vi "ASI_stage_main.vi"   [LabVIEW 2015]
uses:
  CONTROLS/Q_main_element.ctl
  CONTROLS/Q_ASI_stage_element.ctl
  GLOBAL/Global_ASI_stage.vi
  GLOBAL/Global_ABORT.vi
  GLOBAL/Global_MAIN.vi
types:
  T1 = typedef "Q_ASI_stage_element.ctl" = cluster{"variant":variant, "Instruction":enum16{"ASI_idle", "ASI_initialize", "ASI_error", "ASI_security_stop", "ASI_read_XYZ", "ASI_up", "ASI_down", "ASI_left", "ASI_right", "ASI_save_XY", "ASI_move_to_XY", "ASI_brightfield", "ASI_init_scan", "ASI_init_merFISH", "ASI_move_to_XY_merFISH", "ASI_move_to_Z_merFISH", "ASI_init_autofocus_search_merFISH", "ASI_close_autofocus_search_merFISH", "ASI_adjust_piezo_autofocus_merFISH", "ASI_set_piezo_autofocus_to_reference_position_merFISH_TL", "ASI_close_merFISH", "ASI_stop"}}
  T2 = typedef "Q_main_element.ctl" = cluster{"variant":variant, "Instruction":enum16{"Main_idle", "Main_initialize", "Main_initialize_TDMS", "Main_initialize_Queue", "Main_error", "Main_DAQ_initialization_results", "Main_ASI_initialization_results", "Main_Piezo_initialization_results", "Main_Valve_initialization_results", "Main_Pump_initialization_results", "Main_CAMERA_initialization_results", "Main_FPGA_initialization_results", "Main_DAQ_error", "Main_ASI_error", "Main_Piezo_error", "Main_CAMERA_error", "Main_Valve_error", "Main_Pump_error", "Main_FPGA_error", "Main_start_acquiring", "Main_not_acquiring", "Main_acquiring", "Main_stop_acquiring", "Main_change_exposure", "Main_change_z_scan_parameters", "Main_define_ROI", "Main_define_mosaic", "Main_read_kinetic_time", "Main_cooler", "Main_read_temperature", "Main_save_XY", "Main_load_XY", "Main_discard_XY", "Main_move_to_XY", "Main_measure_QPD", "Main_autofocus_calibration", "Main_autofocus_initialization", "Main_autofocus_stop", "Main_save_PID", "Main_change_H_valve_position", "Main_two_way_valve", "Main_save_movie", "Main_init_single_scan", "Main_single_scan", "Main_stop_single_scan", "Main_merFISH_illumination_parameters", "Main_merFISH_buffer_probe_list", "Main_merFISH_injections_procedure", "Main_merFISH_save_setpoint", "Main_merFISH_DAPI_parameters", "Main_merFISH_Brightfield_parameters", "Main_merFISH_save_embryo_ROI", "Main_merFISH_init", "Main_merFISH_resume", "Main_merFISH_start_autofocus", "Main_merFISH_open_close_valve_merFISH", "Main_merFISH_open_close_valve_photobleaching", "Main_merFISH_hybridization", "Main_merFISH_move_to_ROI", "Main_merFISH_wait_stabilization", "Main_merFISH_move_to_REF", "Main_merFISH_scan", "Main_merFISH_photobleaching_injection", "Main_merFISH_photobleaching", "Main_merFISH_send_email", "Main_merFISH_close", "Main_STOP"}}
  T3 = cluster{"XY ROI0":dbl[], "Brightfield intensity":dbl, "Illumination source":bool}
  T4 = enum16{"ASI_idle", "ASI_initialize", "ASI_error", "ASI_security_stop", "ASI_read_XYZ", "ASI_up", "ASI_down", "ASI_left", "ASI_right", "ASI_save_XY", "ASI_move_to_XY", "ASI_brightfield", "ASI_init_scan", "ASI_init_merFISH", "ASI_move_to_XY_merFISH", "ASI_move_to_Z_merFISH", "ASI_init_autofocus_search_merFISH", "ASI_close_autofocus_search_merFISH", "ASI_adjust_piezo_autofocus_merFISH", "ASI_set_piezo_autofocus_to_reference_position_merFISH_TL", "ASI_close_merFISH", "ASI_stop"}
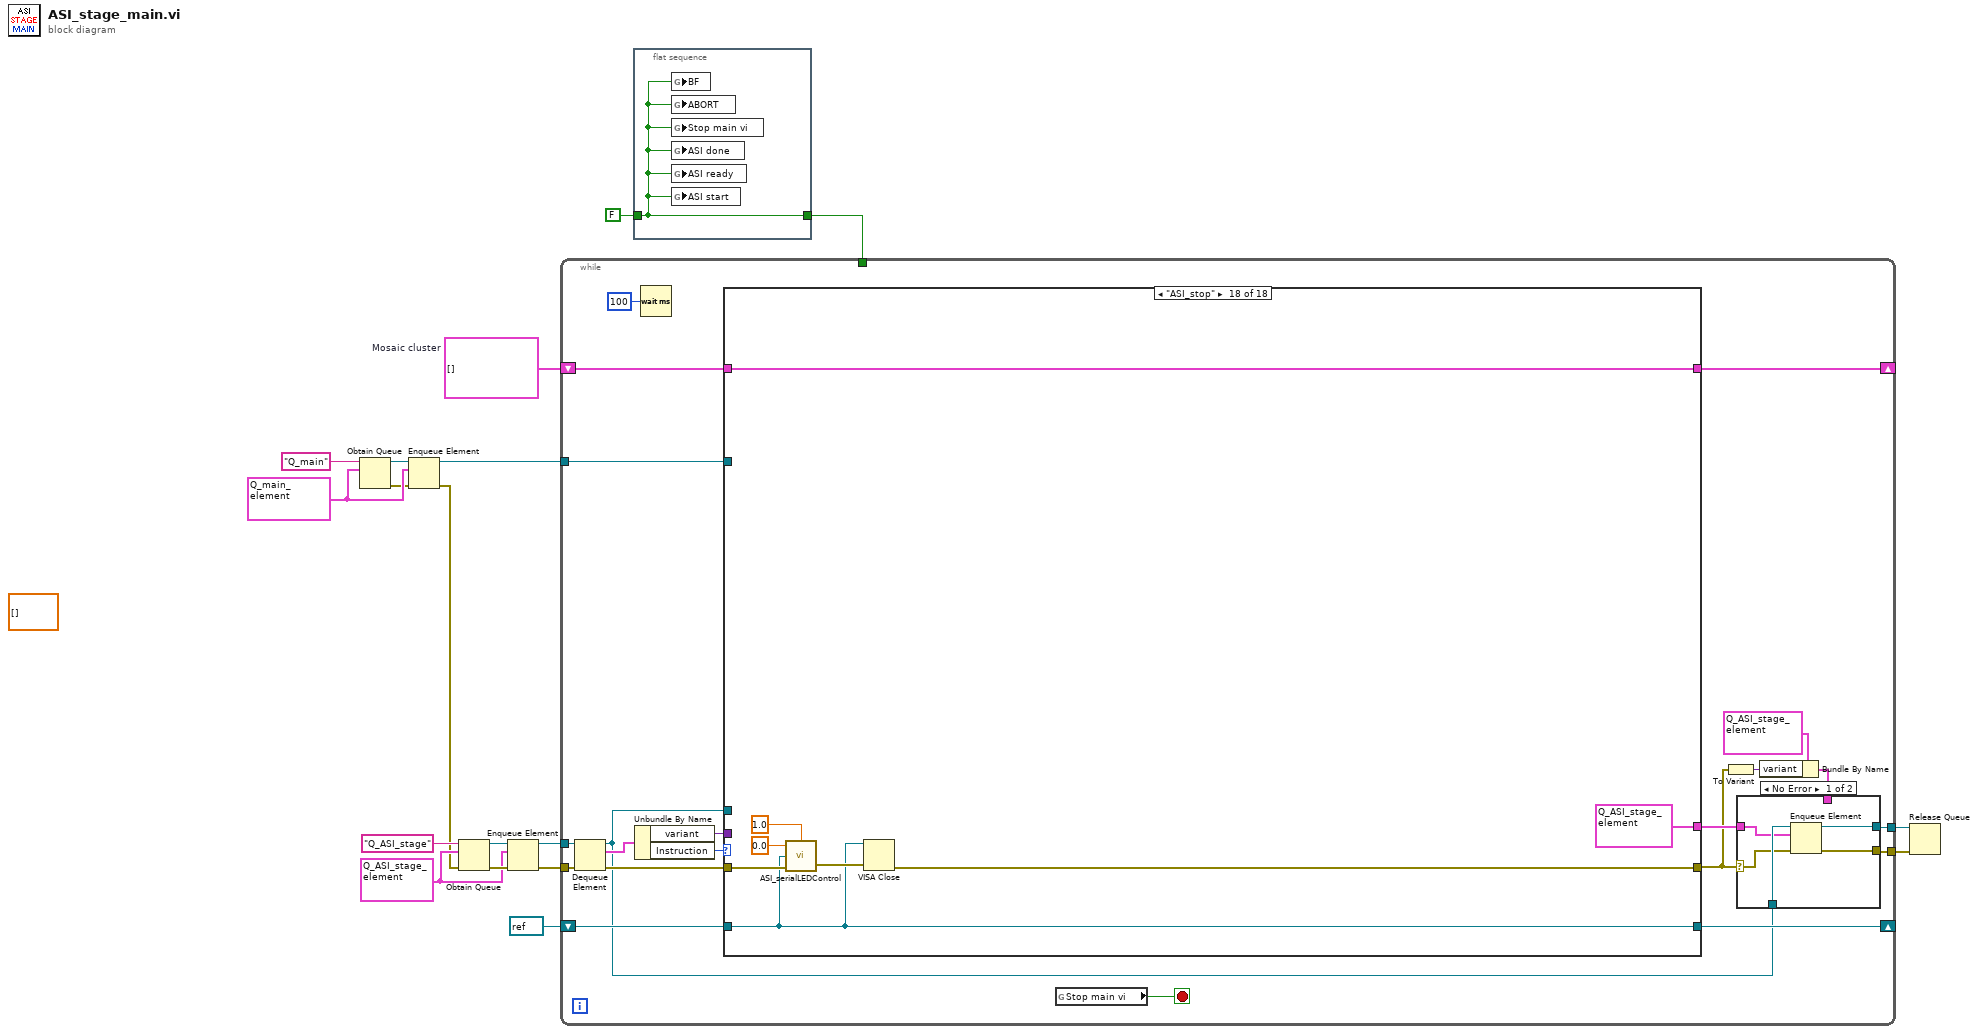
[diagram p0: block diagram]
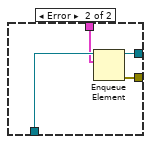
[diagram p2: hidden frame]
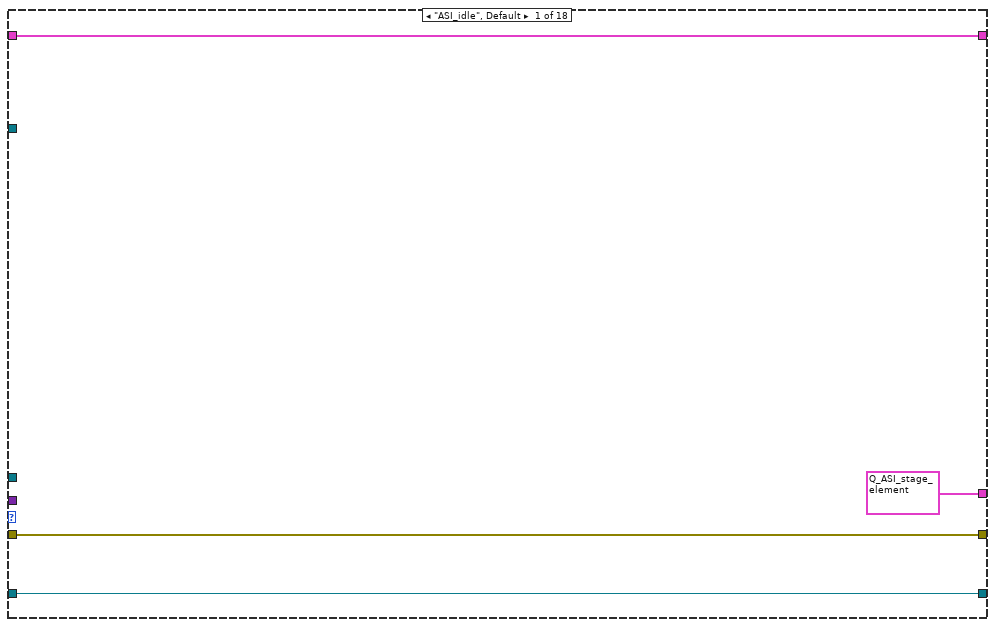
[diagram p3: hidden frame]
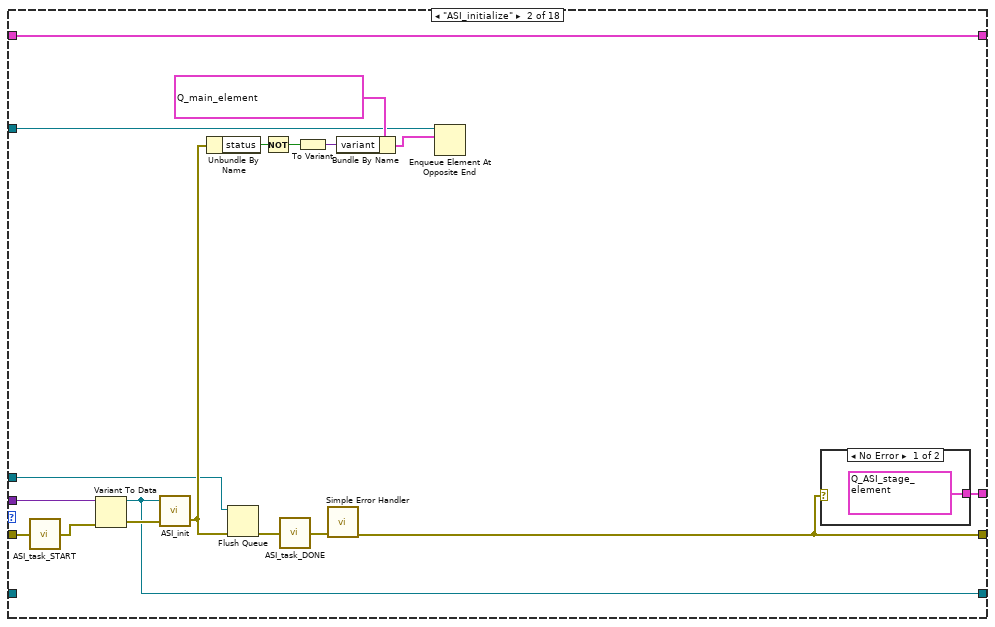
[diagram p4: hidden frame]
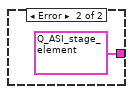
[diagram p5: hidden frame]
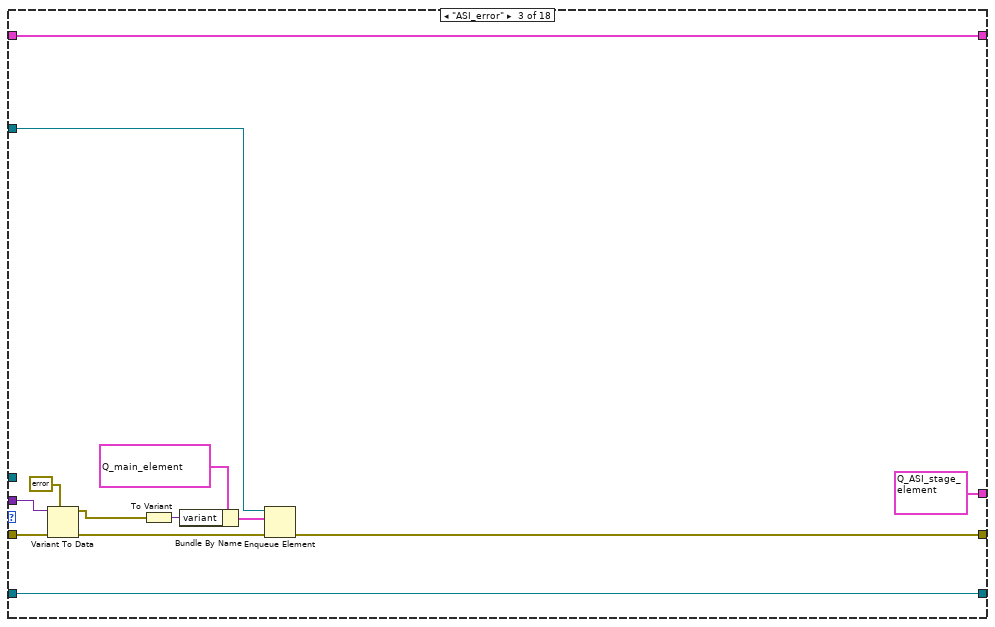
[diagram p6: hidden frame]
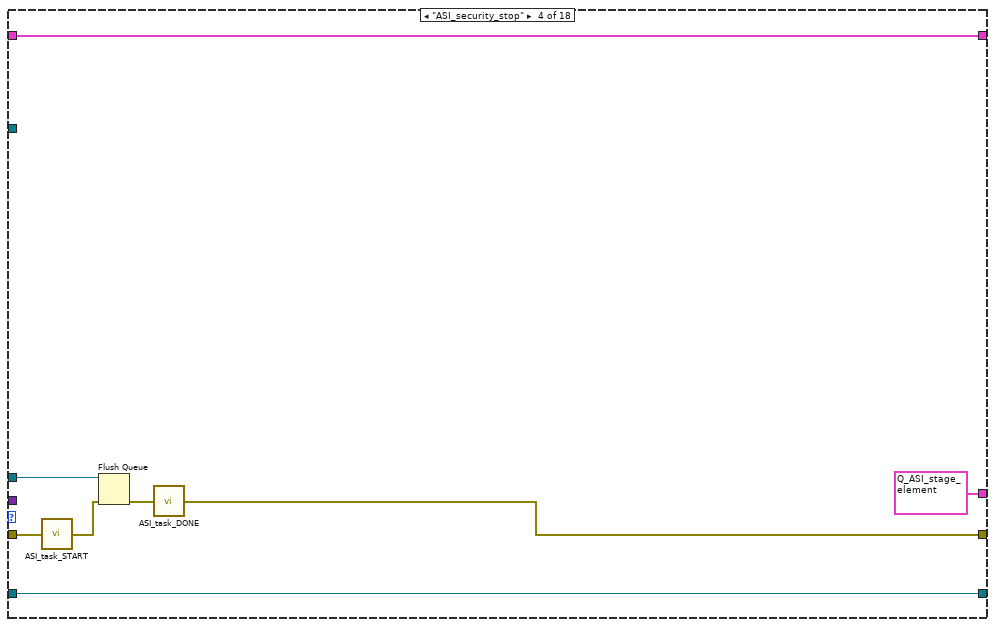
[diagram p7: hidden frame]
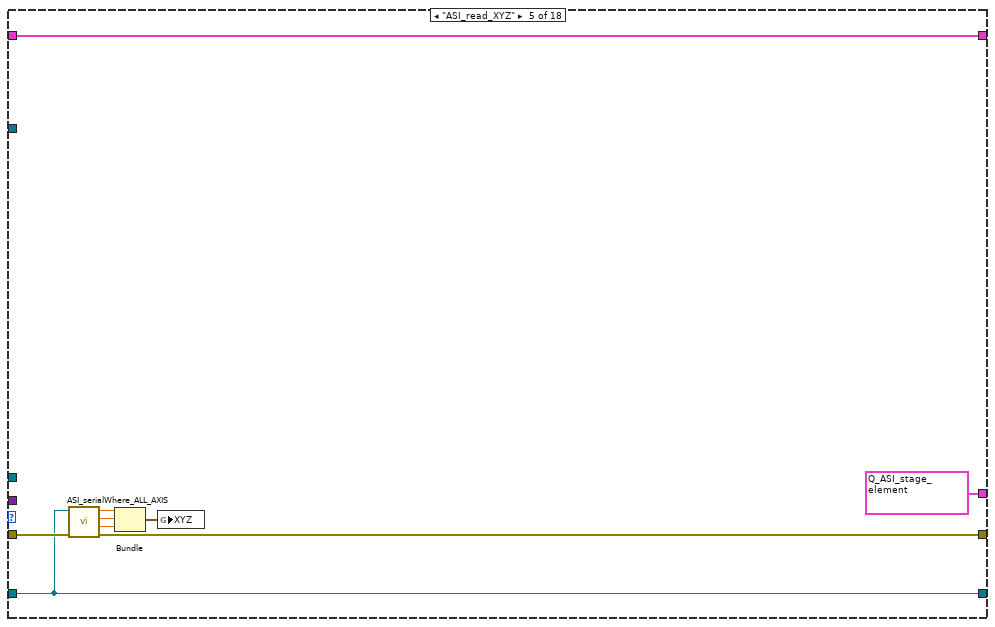
[diagram p8: hidden frame]
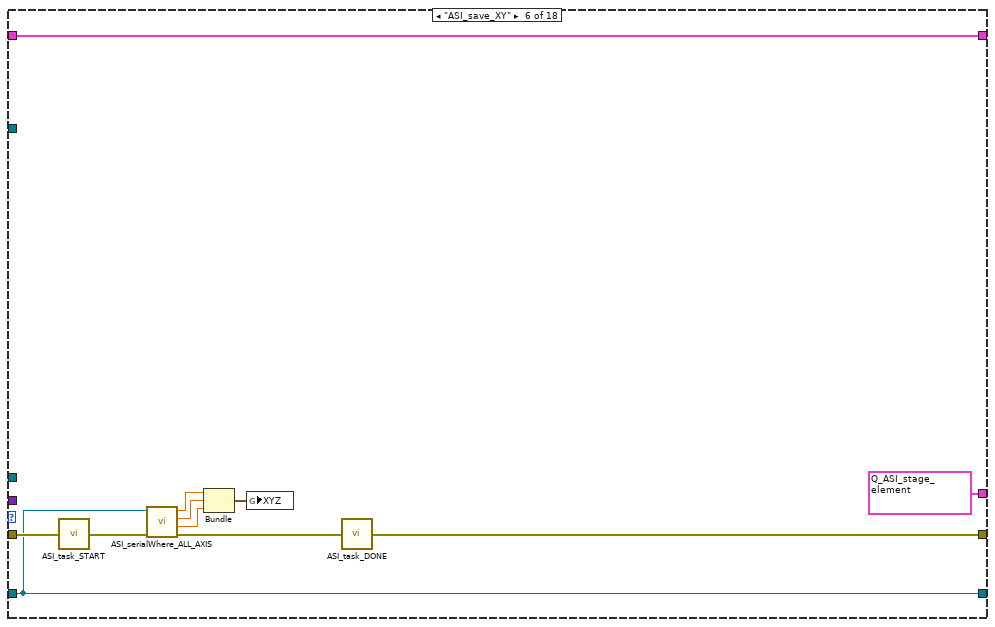
[diagram p9: hidden frame]
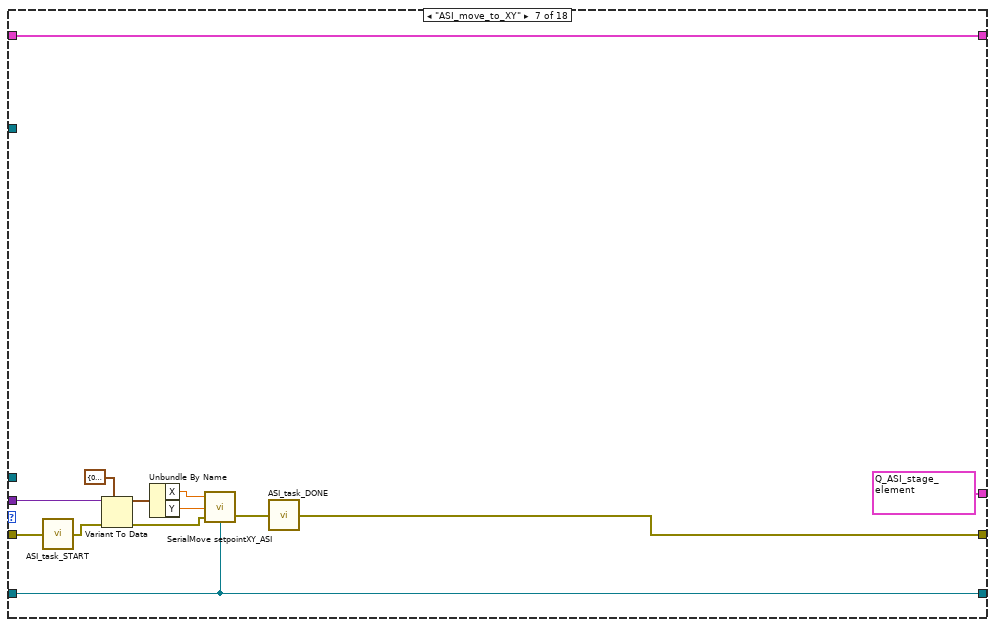
[diagram p10: hidden frame]
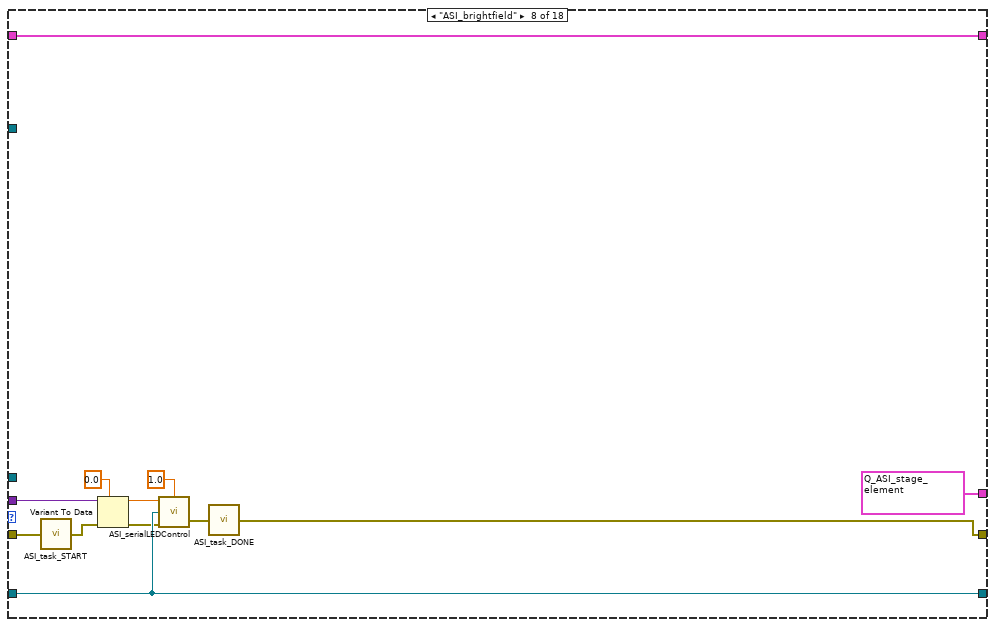
[diagram p11: hidden frame]
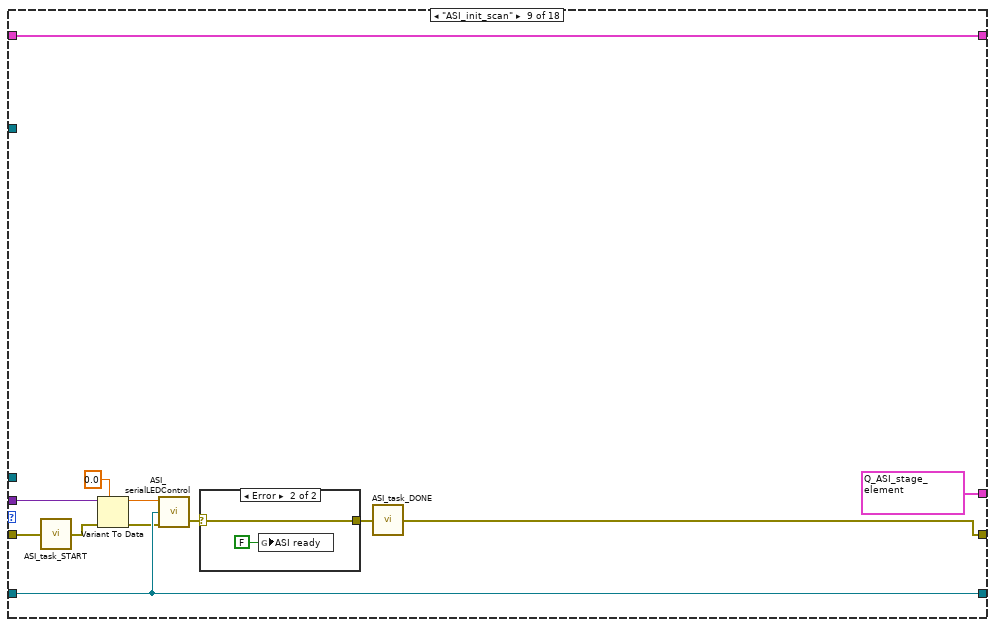
[diagram p12: hidden frame]
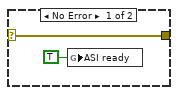
[diagram p13: hidden frame]
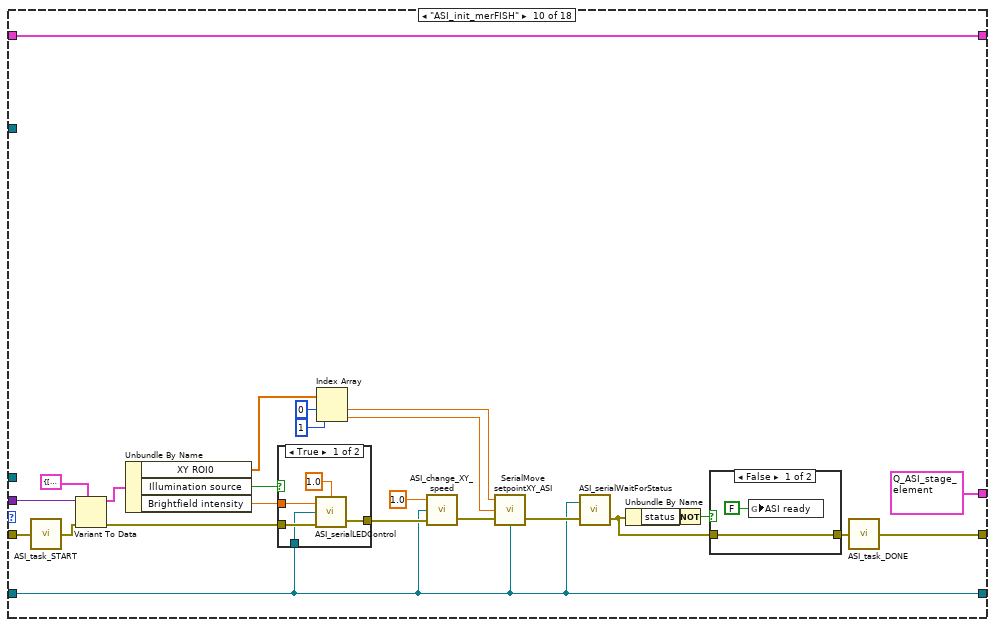
[diagram p14: hidden frame]
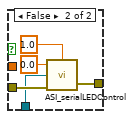
[diagram p15: hidden frame]
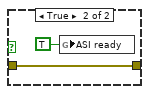
[diagram p16: hidden frame]
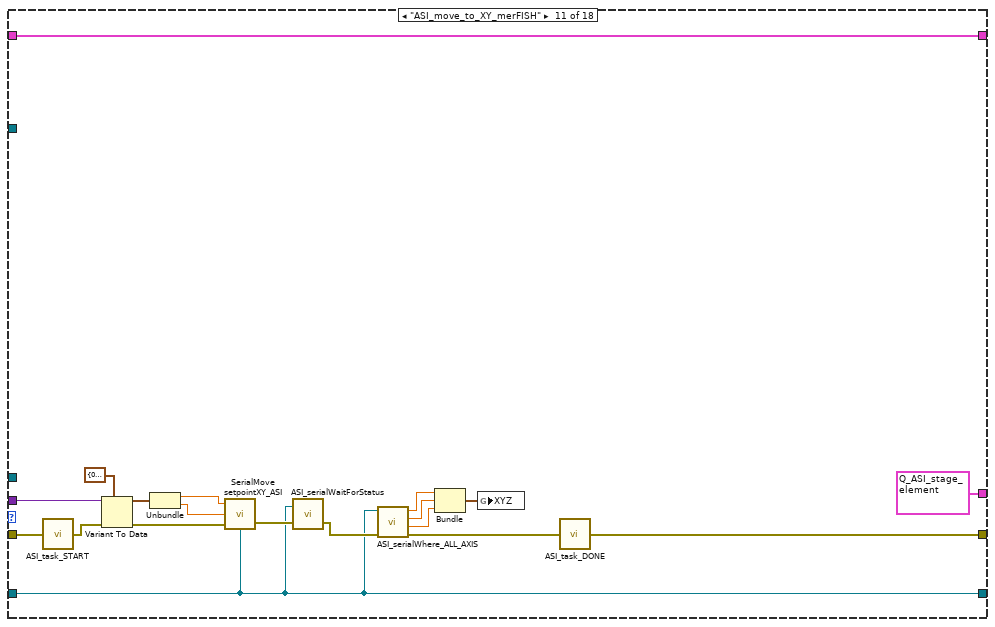
[diagram p17: hidden frame]
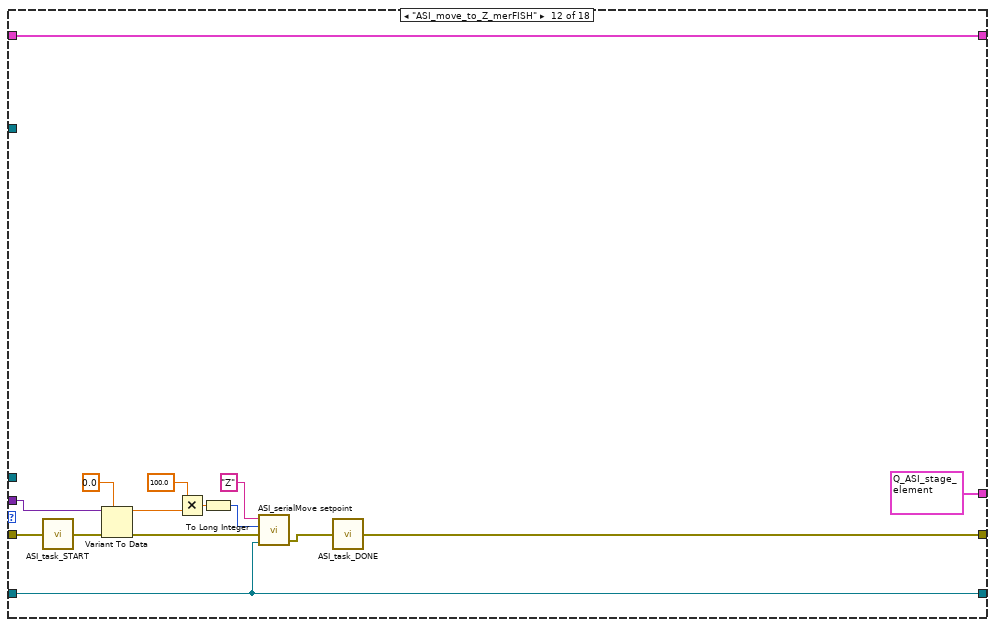
[diagram p18: hidden frame]
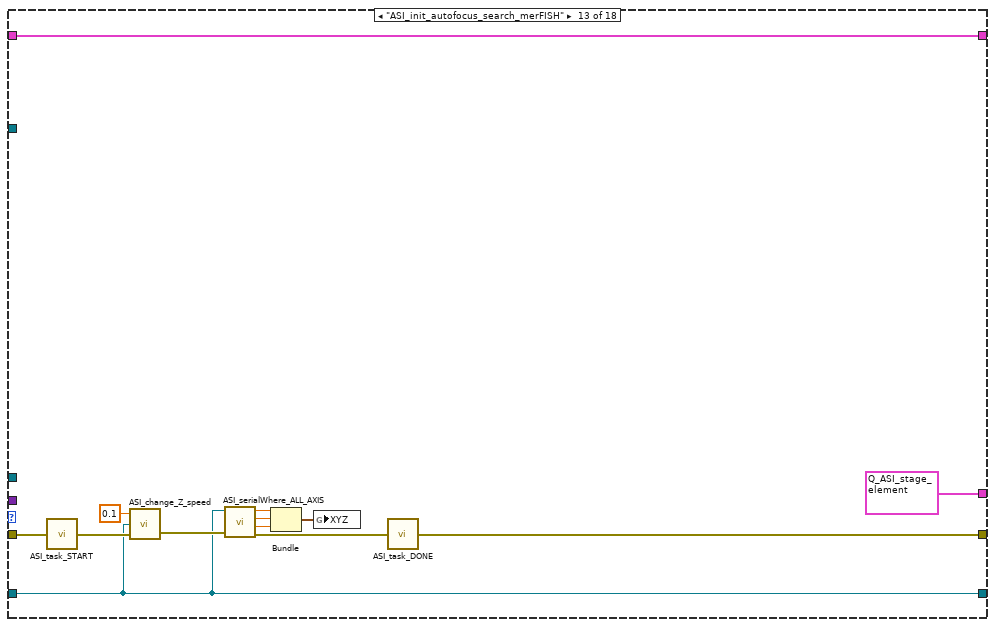
[diagram p19: hidden frame]
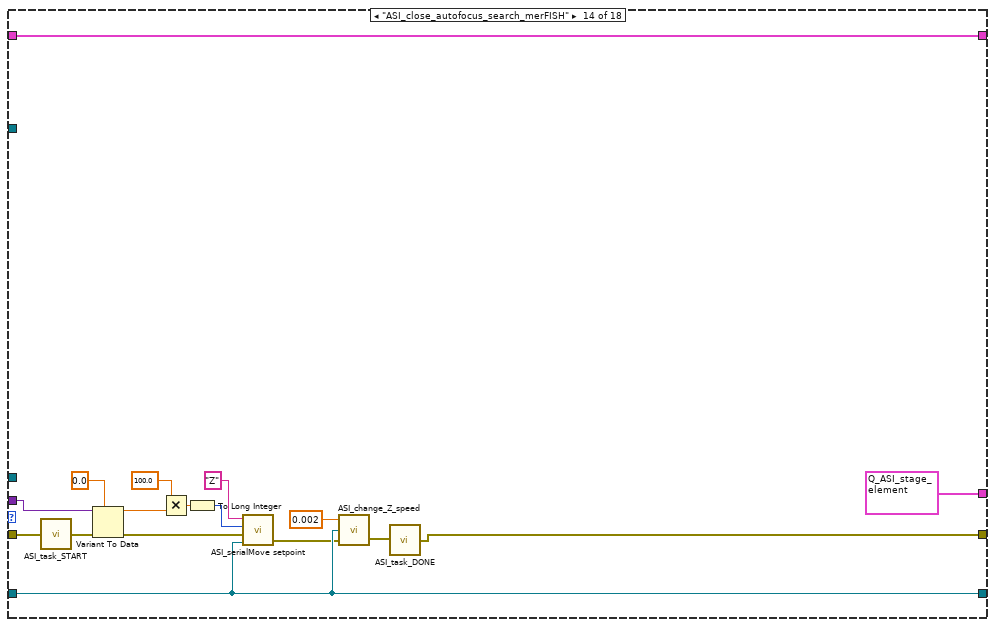
[diagram p20: hidden frame]
diagram:
  w1 = cluster{dbl[], dbl[]}[] []  # Mosaic cluster
  (unwired) dbl[][] [] ("XY positions 2")
  w4 = T1 {"variant"=variant, "Instruction"=enum."ASI_idle"} ("Q_ASI_stage")
  w11 = T2 {"variant"=variant, "Instruction"=enum."Main_idle"} ("Q_main_element")
  n1 = Obtain Queue(name (unnamed)="Q_main", element data type=w11) -> (queue out=w9:refnum<queue>, error out=w10:errorcluster)  [unwired: 3 in, 1 out]
  n2 = Enqueue Element(queue=w9, element=w11, error in (no error)=w10) -> (queue out=w7:refnum<queue>, error out=w2:errorcluster)  [unwired: 1 in, 1 out]
  n3 = Obtain Queue(name (unnamed)="Q_ASI_stage", element data type=w4, error in (no error)=w2) -> (queue out=w17:refnum<queue>, error out=w16:errorcluster)  [unwired: 2 in, 1 out]
  n4 = Enqueue Element(queue=w17, element=w4, error in (no error)=w16) -> (queue out=w15:refnum<queue>, error out=w14:errorcluster)  [unwired: 1 in, 1 out]
  n5 = while {
    tunnel: w15 -> [w38]
    tunnel: w14 -> [w37]
    tunnel: [w32] -> w13
    tunnel: [w31] -> w12
    tunnel: w7 -> [w30]
    tunnel: w5 -> [_]
    shift-right: [w26] -> _
    shift-left: refnum<visa-resource-name> refnum ("VISA resource name") -> [w27]
    shift-right: [w21] -> _
    shift-left: w1 -> [w20]
    stop <- w39 stop-if-true
    n6 = Dequeue Element(queue=w38, error in (no error)=w37) -> (queue out=w19:refnum<queue>, element=w36:T1, error out=w34:errorcluster)  [unwired: 1 in, 1 out]
    n7 = Unbundle By Name(w36) -> ("variant"=w29:variant, "Instruction"=w35:T4)
    n8 = Wait (ms)(milliseconds to wait=u32 100) -> ()  [unwired: 1 out]
    n9 = case shown="\"ASI_stop\"" w35 {
      tunnel: w34 -> [w52 w68 w80 w91 w102 w113 w126 w137 w149 w178 w212 w215 w240 w247 w262 w303 w331 w339]
      tunnel: [w52 w54 w74 w88 w101 w108 w121 w130 w142 w174 w207 w214 w234 w256 w259 w300 w330 w340] -> w22
      tunnel: [T1 {"variant"=variant, "Instruction"=enum."ASI_idle"} ("Q_ASI_stage") w70 T1 {"variant"=variant, "Instruction"=enum."ASI_idle"} ("Q_ASI_stage") T1 {"variant"=variant, "Instruction"=enum."ASI_idle"} ("Q_ASI_stage") T1 {"variant"=variant, "Instruction"=enum."ASI_read_XYZ"} ("Q_ASI_stage") T1 {"variant"=variant, "Instruction"=enum."ASI_read_XYZ"} ("Q_ASI_stage") T1 {"variant"=variant, "Instruction"=enum."ASI_read_XYZ"} ("Q_ASI_stage") T1 {"variant"=variant, "Instruction"=enum."ASI_read_XYZ"} ("Q_ASI_stage") T1 {"variant"=variant, "Instruction"=enum."ASI_read_XYZ"} ("Q_ASI_stage") T1 {"variant"=variant, "Instruction"=enum."ASI_idle"} ("Q_ASI_stage") T1 {"variant"=variant, "Instruction"=enum."ASI_idle"} ("Q_ASI_stage") T1 {"variant"=variant, "Instruction"=enum."ASI_idle"} ("Q_ASI_stage") T1 {"variant"=variant, "Instruction"=enum."ASI_idle"} ("Q_ASI_stage") T1 {"variant"=variant, "Instruction"=enum."ASI_idle"} ("Q_ASI_stage") T1 {"variant"=variant, "Instruction"=enum."ASI_idle"} ("Q_ASI_stage") T1 {"variant"=variant, "Instruction"=enum."ASI_idle"} ("Q_ASI_stage") T1 {"variant"=variant, "Instruction"=enum."ASI_read_XYZ"} ("Q_ASI_stage") T1 {"variant"=variant, "Instruction"=enum."ASI_stop"} ("Q_ASI_stage")] -> w33
      tunnel: w30 -> [_ w63 w77 _ _ _ _ _ _ _ _ _ _ _ _ _ _ _]
      tunnel: w29 -> [_ w69 w81 _ _ _ w125 w138 w150 w179 w211 w227 _ w246 w261 w304 _ _]
      tunnel: w19 -> [_ w57 _ w90 _ _ _ _ _ _ _ _ _ _ _ _ _ _]
      tunnel: w27 -> [w50 _ w84 w92 w99 w112 w116 w135 w147 w162 w195 w217 w230 w249 w260 w302 w326 w337]
      tunnel: [w50 w60 w84 w92 w99 w112 w116 w135 w147 w162 w195 w217 w230 w249 w260 w302 w326 w337] -> w26
      tunnel: [w49 w53 w73 w86 w94 w103 w114 w128 w139 w159 w194 w213 w228 w241 w258 w298 w321 w335] -> w21
      tunnel: w20 -> [w49 w53 w73 w86 w94 w103 w114 w128 w139 w159 w194 w213 w228 w241 w258 w298 w321 w335]
      frame "ASI_idle", Default {
      }
      frame "ASI_initialize" {
        n10 = call "ASI_task_START.vi"("error in"=w68) -> ("error out"=w56:errorcluster)
        n11 = Variant To Data(error in=w56, Variant=w69) -> (data=w60:refnum<visa-resource-name>, error out=w67:errorcluster)  [unwired: 1 in]
        n12 = call "ASI_init.vi"("error in (no error)"=w67, "VISA resource name"=w60) -> ("error out"=w59:errorcluster)  [unwired: 1 in, 1 out]
        n13 = Unbundle By Name(w59) -> ("status"=w62:bool)
        n14 = Flush Queue(queue=w57, error in (no error)=w59) -> (error out=w58:errorcluster)  [unwired: 2 out]
        n15 = Not(x=w62) -> (.not. x?=w61:bool)
        n16 = call "ASI_task_DONE.vi"("error in"=w58) -> ("error out"=w55:errorcluster)
        n17 = To Variant(anything=w61) -> (Variant=w65:variant)
        n18 = call <vilib>:"Simple Error Handler.vi"("error in (no error)"=w55) -> ("error out"=w54:errorcluster)  [unwired: 4 in, 4 out]
        n19 = Bundle By Name(cluster=T2 {"variant"=variant, "Instruction"=enum."Main_ASI_initialization_results"} ("element"), "variant"=w65) -> (w66:T2)
        n20 = Enqueue Element At Opposite End(queue=w63, element=w66) -> ()  [unwired: 2 in, 3 out]
        n21 = case shown="No Error" w54 {
          tunnel: [T1 {"variant"=variant, "Instruction"=enum."ASI_read_XYZ"} ("Q_ASI_stage") T1 {"variant"=variant, "Instruction"=enum."ASI_idle"} ("Q_ASI_stage")] -> w70
          frame No Error {
          }
          frame Error {
          }
        }
      }
      frame "ASI_error" {
        n22 = Variant To Data(error in=w80, type=errorcluster {"status"=FALSE, "code"=0, "source"=""} ("error out"), Variant=w81) -> (data=w75:errorcluster, error out=w76:errorcluster)
        n23 = To Variant(anything=w75) -> (Variant=w82:variant)
        n24 = Bundle By Name(cluster=T2 {"variant"=variant, "Instruction"=enum."Main_ASI_error"} ("Q_main_element"), "variant"=w82) -> (w78:T2)
        n25 = Enqueue Element(queue=w77, element=w78, error in (no error)=w76) -> (error out=w74:errorcluster)  [unwired: 1 in, 2 out]
      }
      frame "ASI_security_stop" {
        n26 = call "ASI_task_START.vi"("error in"=w91) -> ("error out"=w89:errorcluster)
        n27 = Flush Queue(queue=w90, error in (no error)=w89) -> (error out=w87:errorcluster)  [unwired: 2 out]
        n28 = call "ASI_task_DONE.vi"("error in"=w87) -> ("error out"=w88:errorcluster)
      }
      frame "ASI_read_XYZ" {
        n29 = call "ASI_serialWhere_ALL_AXIS.vi"("error in (no error)"=w102, "VISA resource name"=w99) -> ("error out"=w101:errorcluster, "Z"=w96:dbl, "Y"=w97:dbl, "X"=w98:dbl)  [unwired: 2 in]
        n30 = Bundle("X"=w98, "Y"=w97, "Z"=w96) -> (w95:cluster{"X":dbl, "Y":dbl, "Z":dbl})  [unwired: 1 in]
        n31 = global write "Global_ASI_stage.vi" "XYZ"(w95) -> ()
      }
      frame "ASI_save_XY" {
        n32 = call "ASI_task_START.vi"("error in"=w113) -> ("error out"=w110:errorcluster)
        n33 = call "ASI_serialWhere_ALL_AXIS.vi"("error in (no error)"=w110, "VISA resource name"=w112) -> ("error out"=w109:errorcluster, "Z"=w105:dbl, "Y"=w106:dbl, "X"=w107:dbl)  [unwired: 2 in]
        n34 = Bundle("X"=w107, "Y"=w106, "Z"=w105) -> (w104:cluster{"X":dbl, "Y":dbl, "Z":dbl})  [unwired: 1 in]
        n35 = global write "Global_ASI_stage.vi" "XYZ"(w104) -> ()
        n36 = call "ASI_task_DONE.vi"("error in"=w109) -> ("error out"=w108:errorcluster)
      }
      frame "ASI_move_to_XY" {
        n37 = call "ASI_task_START.vi"("error in"=w126) -> ("error out"=w124:errorcluster)
        n38 = Variant To Data(error in=w124, type=cluster{"X":dbl, "Y":dbl} {"X"=0.0, "Y"=0.0} ("output cluster"), Variant=w125) -> (data=w122:cluster{"X":dbl, "Y":dbl}, error out=w117:errorcluster)
        n39 = Unbundle By Name(w122) -> ("X"=w119:dbl, "Y"=w118:dbl)
        n40 = call "SerialMove setpointXY_ASI.vi"("VISA resource name"=w116, "error in"=w117, "Y"=w118, "X"=w119) -> ("error out"=w115:errorcluster)  [unwired: 1 in]
        n41 = call "ASI_task_DONE.vi"("error in"=w115) -> ("error out"=w121:errorcluster)
      }
      frame "ASI_brightfield" {
        n42 = call "ASI_task_START.vi"("error in"=w137) -> ("error out"=w131:errorcluster)
        n43 = Variant To Data(error in=w131, type=0.0 ("BF"), Variant=w138) -> (data=w132:dbl, error out=w133:errorcluster)
        n44 = call "ASI_serialLEDControl.vi"("Delay Time (s)"=1.0, "error in (no error)"=w133, "VISA resource name"=w135, "setpoint"=w132) -> ("error out"=w129:errorcluster)  [unwired: 1 out]
        n45 = call "ASI_task_DONE.vi"("error in"=w129) -> ("error out"=w130:errorcluster)
      }
      frame "ASI_init_scan" {
        n46 = call "ASI_task_START.vi"("error in"=w149) -> ("error out"=w143:errorcluster)
        n47 = Variant To Data(error in=w143, type=0.0 ("BF"), Variant=w150) -> (data=w144:dbl, error out=w145:errorcluster)
        n48 = call "ASI_serialLEDControl.vi"("error in (no error)"=w145, "VISA resource name"=w147, "setpoint"=w144) -> ("error out"=w141:errorcluster)  [unwired: 1 in, 1 out]
        n49 = case shown="Error" w141 {
          selector: w141 -> [w152 w154]
          tunnel: [w152 w154] -> w140
          frame No Error {
            n50 = global write "Global_ASI_stage.vi" "ASI ready"(TRUE ("ASI ready")) -> ()
          }
          frame Error {
            n51 = global write "Global_ASI_stage.vi" "ASI ready"(FALSE ("ASI ready")) -> ()
          }
        }
        n52 = call "ASI_task_DONE.vi"("error in"=w140) -> ("error out"=w142:errorcluster)
      }
      frame "ASI_init_merFISH" {
        n53 = call "ASI_task_START.vi"("error in"=w178) -> ("error out"=w175:errorcluster)
        n54 = Variant To Data(error in=w175, type=T3 {"XY ROI0"=[], "Brightfield intensity"=0.0, "Illumination source"=FALSE} ("output cluster"), Variant=w179) -> (data=w172:T3, error out=w176:errorcluster)
        n55 = Unbundle By Name(w172) -> ("XY ROI0"=w156:dbl[], "Illumination source"=w155:bool, "Brightfield intensity"=w171:dbl)
        n56 = case shown="True" w155 {
          tunnel: w176 -> [w184 w189]
          tunnel: w171 -> [w183 _]
          tunnel: [w182 w188] -> w166
          tunnel: w162 -> [w181 w187]
          frame True {
            n57 = call "ASI_serialLEDControl.vi"("Delay Time (s)"=1.0, "error in (no error)"=w184, "VISA resource name"=w181, "setpoint"=w183) -> ("error out"=w182:errorcluster)  [unwired: 1 out]
          }
          frame False {
            n58 = call "ASI_serialLEDControl.vi"("Delay Time (s)"=1.0, "error in (no error)"=w189, "VISA resource name"=w187, "setpoint"=0.0) -> ("error out"=w188:errorcluster)  [unwired: 1 out]
          }
        }
        n59 = Index Array(array=w156, index #1=0 ("index"), index #2=1 ("index")) -> (element #1=w168:dbl, element #2=w167:dbl)
        n60 = call "ASI_change_XY_speed.vi"("error in (no error)"=w166, "VISA resource name"=w162, "speed"=1.0) -> ("error out"=w164:errorcluster)  [unwired: 1 in]
        n61 = call "SerialMove setpointXY_ASI.vi"("VISA resource name"=w162, "error in"=w164, "Y"=w167, "X"=w168) -> ("error out"=w163:errorcluster)  [unwired: 1 in]
        n62 = call "ASI_serialWaitForStatus.vi"("error in"=w163, "VISA resource name"=w162) -> ("error out"=w160:errorcluster)  [unwired: 1 in]
        n63 = Unbundle By Name(w160) -> ("status"=w161:bool)
        n64 = Not(x=w161) -> (.not. x?=w158:bool)
        n65 = case shown="False" w158 {
          tunnel: [w190 w192] -> w173
          tunnel: w160 -> [w190 w192]
          frame False {
            n66 = global write "Global_ASI_stage.vi" "ASI ready"(FALSE ("ASI ready")) -> ()
          }
          frame True {
            n67 = global write "Global_ASI_stage.vi" "ASI ready"(TRUE ("ASI ready")) -> ()
          }
        }
        n68 = call "ASI_task_DONE.vi"("error in"=w173) -> ("error out"=w174:errorcluster)
      }
      frame "ASI_move_to_XY_merFISH" {
        n69 = call "ASI_task_START.vi"("error in"=w212) -> ("error out"=w210:errorcluster)
        n70 = Variant To Data(error in=w210, type=cluster{dbl, dbl} {0.0, 0.0} ("output cluster"), Variant=w211) -> (data=w208:cluster{dbl, dbl}, error out=w200:errorcluster)
        n71 = Unbundle(w208) -> (w198:dbl, w199:dbl)
        n72 = call "SerialMove setpointXY_ASI.vi"("VISA resource name"=w195, "error in"=w200, "Y"=w199, "X"=w198) -> ("error out"=w197:errorcluster)  [unwired: 1 in]
        n73 = call "ASI_serialWaitForStatus.vi"("error in"=w197, "VISA resource name"=w195) -> ("error out"=w196:errorcluster)  [unwired: 1 in]
        n74 = call "ASI_serialWhere_ALL_AXIS.vi"("error in (no error)"=w196, "VISA resource name"=w195) -> ("error out"=w205:errorcluster, "Z"=w202:dbl, "Y"=w203:dbl, "X"=w204:dbl)  [unwired: 2 in]
        n75 = Bundle("X"=w204, "Y"=w203, "Z"=w202) -> (w201:cluster{"X":dbl, "Y":dbl, "Z":dbl})  [unwired: 1 in]
        n76 = global write "Global_ASI_stage.vi" "XYZ"(w201) -> ()
        n77 = call "ASI_task_DONE.vi"("error in"=w205) -> ("error out"=w207:errorcluster)
      }
      frame "ASI_move_to_Z_merFISH" {
        n78 = call "ASI_task_START.vi"("error in"=w215) -> ("error out"=w226:errorcluster)
        n79 = Variant To Data(error in=w226, type=0.0, Variant=w227) -> (data=w218:dbl, error out=w219:errorcluster)
        n80 = Multiply(x=100.0, y=w218) -> (x*y=w221:dbl)
        n81 = To Long Integer(number=w221) -> (32bit integer=w220:i32)
        n82 = call "ASI_serialMove setpoint.vi"("Axis"="Z", "setpoint"=w220, "error in (no error)"=w219, "VISA resource name"=w217) -> ("error out"=w216:errorcluster)  [unwired: 3 in]
        n83 = call "ASI_task_DONE.vi"("error in"=w216) -> ("error out"=w214:errorcluster)
      }
      frame "ASI_init_autofocus_search_merFISH" {
        n84 = call "ASI_task_START.vi"("error in"=w240) -> ("error out"=w232:errorcluster)
        n85 = call "ASI_change_Z_speed.vi"("error in (no error)"=w232, "VISA resource name"=w230, "speed"=0.1) -> ("error out"=w231:errorcluster)  [unwired: 1 out]
        n86 = call "ASI_serialWhere_ALL_AXIS.vi"("error in (no error)"=w231, "VISA resource name"=w230) -> ("error out"=w233:errorcluster, "Z"=w236:dbl, "Y"=w237:dbl, "X"=w238:dbl)  [unwired: 2 in]
        n87 = Bundle("X"=w238, "Y"=w237, "Z"=w236) -> (w235:cluster{"X":dbl, "Y":dbl, "Z":dbl})  [unwired: 1 in]
        n88 = global write "Global_ASI_stage.vi" "XYZ"(w235) -> ()
        n89 = call "ASI_task_DONE.vi"("error in"=w233) -> ("error out"=w234:errorcluster)
      }
      frame "ASI_close_autofocus_search_merFISH" {
        n90 = call "ASI_task_START.vi"("error in"=w247) -> ("error out"=w242:errorcluster)
        n91 = Variant To Data(error in=w242, type=0.0 ("x"), Variant=w246) -> (data=w244:dbl, error out=w243:errorcluster)
        n92 = Multiply(x=100.0, y=w244) -> (x*y=w251:dbl)
        n93 = To Long Integer(number=w251) -> (32bit integer=w250:i32)
        n94 = call "ASI_serialMove setpoint.vi"("Axis"="Z", "setpoint"=w250, "error in (no error)"=w243, "VISA resource name"=w249) -> ("error out"=w248:errorcluster)  [unwired: 3 in]
        n95 = call "ASI_change_Z_speed.vi"("error in (no error)"=w248, "VISA resource name"=w249, "speed"=0.002) -> ("error out"=w254:errorcluster)  [unwired: 1 out]
        n96 = call "ASI_task_DONE.vi"("error in"=w254) -> ("error out"=w256:errorcluster)
      }
      frame "ASI_adjust_piezo_autofocus_merFISH" {
        # "In order to adjust the piezo position to 20um (when piezo position is below 10um)\nor 60um (when it is above 70um) without loosing the focus, \nthe ASI z position is changed here. Since the speed of the ASI stage movement\nis usually too fast, it is set to 2um/s and the backlash set to 1um."
        n97 = call "ASI_task_START.vi"("error in"=w262) -> ("error out"=w265:errorcluster)
        n98 = Variant To Data(error in=w265, type=cluster{"Min":dbl, "Max":dbl, "z":dbl} {"Min"=0.0, "Max"=0.0, "z"=0.0} ("Limits"), Variant=w261) -> (data=w269:cluster{"Min":dbl, "Max":dbl, "z":dbl}, error out=w263:errorcluster)
        n99 = Unbundle By Name(w269) -> ("Min"=w268:dbl, "z"=w267:dbl)
        n100 = Greater?(x=w268, y=w267) -> (0:w264:bool)
        n101 = case shown="True" w264 {
          tunnel: [w272 w285] -> w270
          tunnel: w260 -> [w281 w294]
          tunnel: w263 -> [w280 w293]
          tunnel: w267 -> [w277 w290]
          tunnel: w269 -> [w276 w287]
          frame True {
            n102 = Unbundle By Name(w276) -> ("Min"=w274:dbl)
            n103 = Add(x=w274, y=5.0) -> (x+y=w275:dbl)
            n104 = Subtract(x=w275, y=w277) -> (x-y=w284:dbl)
            n105 = Multiply(x=100.0, y=w284) -> (x*y=w279:dbl)
            n106 = To Long Integer(number=w279) -> (32bit integer=w278:i32)
            n107 = call "ASI_serialRelativeMove setpoint.vi"("VISA resource name"=w281, "error in (no error)"=w280, "setpoint"=w278, "Axis"="Z") -> ("error out"=w272:errorcluster)  [unwired: 1 in]
          }
          frame False {
            n108 = Unbundle By Name(w287) -> ("Max"=w289:dbl)
            n109 = Subtract(x=w289, y=5.0) -> (x-y=w286:dbl)
            n110 = Subtract(x=w286, y=w290) -> (x-y=w297:dbl)
            n111 = Multiply(x=100.0, y=w297) -> (x*y=w292:dbl)
            n112 = To Long Integer(number=w292) -> (32bit integer=w291:i32)
            n113 = call "ASI_serialRelativeMove setpoint.vi"("VISA resource name"=w294, "error in (no error)"=w293, "setpoint"=w291, "Axis"="Z") -> ("error out"=w285:errorcluster)  [unwired: 1 in]
          }
        }
        n114 = call "ASI_task_DONE.vi"("error in"=w270) -> ("error out"=w259:errorcluster)
      }
      frame "ASI_set_piezo_autofocus_to_reference_position_merFISH_TL" {
        # "In order to adjust the piezo position to 20um (when piezo position is below 10um)\nor 60um (when it is above 70um) without loosing the focus, \nthe ASI z position is changed here. Since the speed of the ASI stage movement\nis usually too fast, it is set to 2um/s and the backlash set to 1um."
        n115 = call "ASI_task_START.vi"("error in"=w303) -> ("error out"=w316:errorcluster)
        n116 = call "ASI_change_Z_speed.vi"("error in (no error)"=w316, "VISA resource name"=w302, "speed"=0.001) -> ("error out"=w299:errorcluster)  [unwired: 1 out]
        n117 = Variant To Data(error in=w299, type=cluster{"Ref":dbl, "z":dbl} {"Ref"=0.0, "z"=0.0} ("Limits"), Variant=w304) -> (data=w308:cluster{"Ref":dbl, "z":dbl}, error out=w305:errorcluster)
        n118 = Unbundle By Name(w308) -> ("Ref"=w314:dbl, "z"=w307:dbl)
        n119 = Subtract(x=w314, y=w307) -> (x-y=w309:dbl)
        n120 = Multiply(x=100.0, y=w309) -> (x*y=w312:dbl)
        n121 = To Long Integer(number=w312) -> (32bit integer=w313:i32)
        n122 = call "ASI_serialRelativeMove setpoint.vi"("VISA resource name"=w302, "error in (no error)"=w305, "setpoint"=w313, "Axis"="Z") -> ("error out"=w317:errorcluster)  [unwired: 1 in]
        n123 = call "ASI_change_Z_speed.vi"("error in (no error)"=w317, "VISA resource name"=w302, "speed"=0.5) -> ("error out"=w318:errorcluster)  [unwired: 1 out]
        n124 = call "ASI_task_DONE.vi"("error in"=w318) -> ("error out"=w300:errorcluster)
      }
      frame "ASI_close_merFISH" {
        n125 = call "ASI_task_START.vi"("error in"=w331) -> ("error out"=w329:errorcluster)
        n126 = call "ASI_serialLEDControl.vi"("Delay Time (s)"=1.0, "error in (no error)"=w329, "VISA resource name"=w326, "setpoint"=0.0) -> ("error out"=w327:errorcluster)  [unwired: 1 out]
        n127 = call "ASI_change_XY_speed.vi"("error in (no error)"=w327, "VISA resource name"=w326, "speed"=7.0) -> ("error out"=w324:errorcluster)  [unwired: 1 in]
        n128 = flat-sequence {
          tunnel: w324 -> [w333]
          tunnel: [w333] -> w323
          frame #0 {
            n129 = global write "Global_ASI_stage.vi" "ASI ready"(FALSE ("ASI ready")) -> ()
          }
        }
        n130 = call "ASI_task_DONE.vi"("error in"=w323) -> ("error out"=w330:errorcluster)
      }
      frame "ASI_stop" {
        n131 = call "ASI_serialLEDControl.vi"("Delay Time (s)"=1.0, "error in (no error)"=w339, "VISA resource name"=w337, "setpoint"=0.0) -> ("error out"=w338:errorcluster)  [unwired: 1 out]
        n132 = VISA Close(VISA resource name=w337, error in (no error)=w338) -> (error out=w340:errorcluster)
      }
    }
    n133 = global read "Global_MAIN.vi" "Stop main vi"() -> (w39:bool)
    n134 = To Variant(anything=w22) -> (Variant=w23:variant)
    n135 = Bundle By Name(cluster=T1 {"variant"=variant, "Instruction"=enum."ASI_error"} ("Q_ASI_stage"), "variant"=w23) -> (w24:T1)
    n136 = case shown="No Error" w22 {
      selector: w22 -> [w41 _]
      tunnel: w33 -> [w40 _]
      tunnel: [w44 w48] -> w32
      tunnel: [w43 w47] -> w31
      tunnel: w19 -> [w42 w46]
      tunnel: w24 -> [_ w45]
      frame No Error {
        n137 = Enqueue Element(queue=w42, element=w40, error in (no error)=w41) -> (queue out=w44:refnum<queue>, error out=w43:errorcluster)  [unwired: 1 in, 1 out]
      }
      frame Error {
        n138 = Enqueue Element(queue=w46, element=w45) -> (queue out=w48:refnum<queue>, error out=w47:errorcluster)  [unwired: 2 in, 1 out]
      }
    }
  }
  n139 = flat-sequence {
    tunnel: FALSE ("Stop main vi") -> [w342]
    tunnel: [w342] -> w5
    frame #0 {
      n140 = global write "Global_ASI_stage.vi" "BF"(w342) -> ()
      n141 = global write "Global_ABORT.vi" "ABORT"(w342) -> ()
      n142 = global write "Global_MAIN.vi" "Stop main vi"(w342) -> ()
      n143 = global write "Global_ASI_stage.vi" "ASI done"(w342) -> ()
      n144 = global write "Global_ASI_stage.vi" "ASI ready"(w342) -> ()
      n145 = global write "Global_ASI_stage.vi" "ASI start"(w342) -> ()
    }
  }
  n146 = Release Queue(queue=w13, error in (no error)=w12) -> ()  [unwired: 1 in, 3 out]
